vi "Create.vi"(8 "error in (no error)":errorcluster, 9 "Configuration File Path":path=path "") -> (0 "error out":errorcluster, 3 "Execution UI Out":refnum<class "Execution UI.lvclass">)   [LabVIEW 2020, in "Execution UI.lvclass"]
uses:
  Execution UI.lvclass
  C:/git/astemes-lunit/source/User Interface/Process/Process.lvclass
  Execution UI.lvclass/Execution UI.ctl
  Process/Process.lvclass
  Result Model/Result Model.lvclass
  Framework/Parallell Test Runner/Parallell Test Runner.lvclass
  C:/git/astemes-lunit/source/User Interface/Execution UI/Execution UI.lvclass
  C:/git/astemes-lunit/source/Core/Result Observer/Result Observer.lvclass
  C:/git/astemes-lunit/source/Framework/Parallell Test Runner/Parallell Test Runner.lvclass
  C:/git/astemes-lunit/source/Framework/Test Runner/Test Runner.lvclass
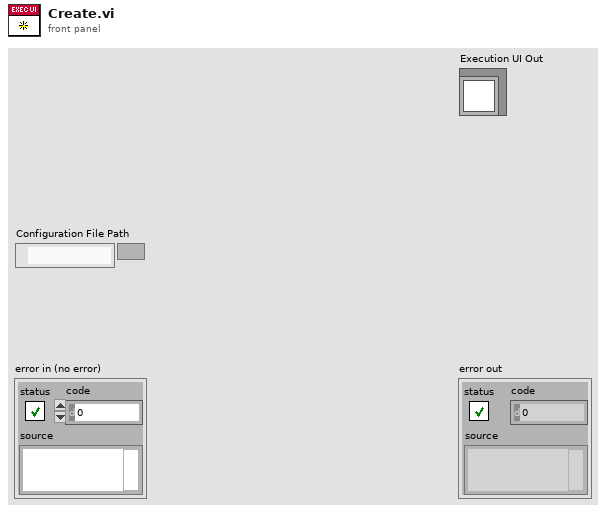
[diagram p1: front panel]
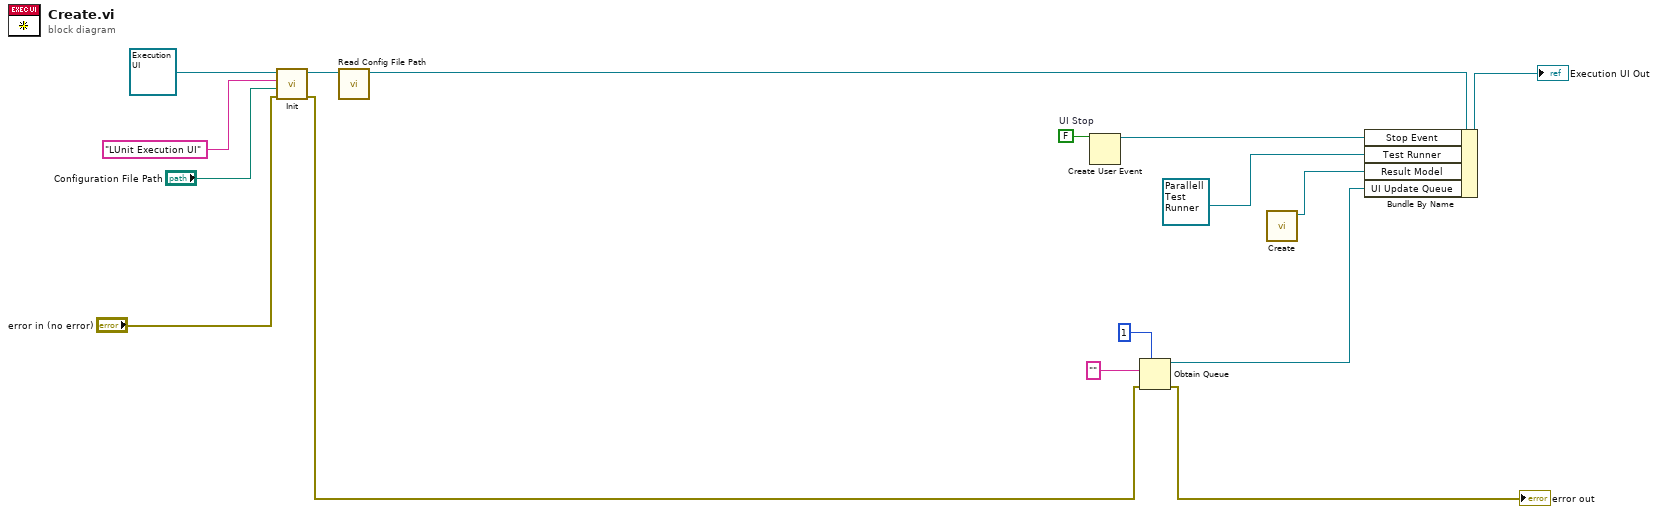
[diagram p0: block diagram]
diagram:
  w11 = FALSE  # UI Stop
  n1 = call-dynamic "Init.vi"("error in (no error)"="error in (no error)", "Config File Path"="Configuration File Path", "Name"="LUnit Execution UI", "Process In"=refnum<class "Execution UI.lvclass"> refnum ("Execution UI In")) -> ("error out"=w2:errorcluster, "Process Out"=w9:refnum<class "Execution UI.lvclass">)  [unwired: 6 in]
  n2 = call "Read Config File Path.vi"("Process In"=w9) -> ("Process Out"=w8:refnum<class "Execution UI.lvclass">)  [unwired: 9 in, 1 out]
  n3 = Create User Event(user event datatype=w11) -> (user event=w10:refnum<user-event>)  [unwired: 1 in, 1 out]
  n4 = Obtain Queue(max queue size (-1, unlimited)=1, element data type="", error in (no error)=w2) -> (queue out=w3:refnum<queue>, error out=→"error out":errorcluster)  [unwired: 2 in, 1 out]
  n5 = call "Create.vi"() -> ("Result Model out"=w6:refnum<class "Result Model.lvclass">)  [unwired: 11 in]
  n6 = Bundle By Name(cluster=w8, "Stop Event"=w10, "Test Runner"=refnum<class "Parallell Test Runner.lvclass"> refnum ("Parallell Test Runner.lvclass"), "Result Model"=w6, "UI Update Queue"=w3) -> (→"Execution UI Out":refnum<class "Execution UI.lvclass">)
